vi "Assign New GUID to Refnum.vi"(8 "error in (no error)":errorcluster, 11 "Item Ref in":T1 format="%.0x") -> (0 "error out":errorcluster, 3 "Item Ref out":T1 format="%.0x")   [LabVIEW 2018, in "Instrument Addon Scripting API.lvlib"]
uses:
  Instrument Addon Scripting API.lvlib
  <vilib>/NI Veristand/Custom Device API/Custom Device Item Ref.ctl
  Addon/Addon Shared/SubVIs/Constants.vi
  <vilib>/NI Veristand/Custom Device API/Set Item Property (String).vi
  Addon/Addon Shared/Instrument Addon Shared.lvlib
  <vilib>/NI Veristand/Custom Device API/Custom Device API.lvlib
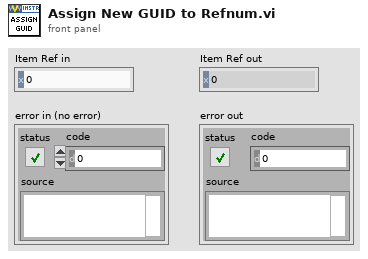
[diagram p1: front panel]
types:
  T1 = typedef "Custom Device API.lvlib/Custom Device Item Ref.ctl" = u64
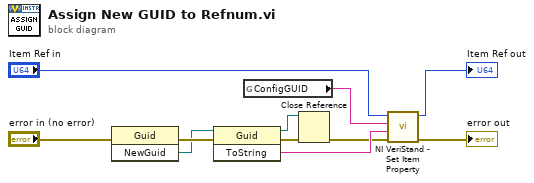
[diagram p0: block diagram]
diagram:
  n1 = invoke class="Guid" method="NewGuid"(error in="error in (no error)") -> (error out=w4:errorcluster, "NewGuid"=w3:refnum<k24>)  [unwired: 2 in, 1 out]
  n2 = invoke class="Guid" method="ToString"(reference=w3, error in=w4) -> (reference out=w2:refnum<k24>, error out=w5:errorcluster, "ToString"=w7:string)  [unwired: 1 in]
  n3 = global read "Constants.vi" "ConfigGUID"() -> (w1:string)
  n4 = Close Reference(reference=w2, error in (no error)=w5) -> (error out=w6:errorcluster)
  n5 = call-poly <vilib>:"NI VeriStand - Set Item Property.vi"("error in (no error)"=w6, "Value"=w7, "Property Name"=w1, "Item Ref in"="Item Ref in") -> ("error out"=→"error out":errorcluster, "Item Ref out"=→"Item Ref out":T1)  [unwired: 5 in, 1 out]
